vi "string2timestamp.vi"(1 "date/time string":string) -> (0 "time stamp":timestamp)   [LabVIEW 2010]
doc: "This VI convert a date/time string back to a time stamp."
uses:
  <vilib>/Utility/miscctls.llb/LVDateTimeRec.ctl
panel:
  # "This control should have data in the form:\n4/30/2004 7:48:47 PM"
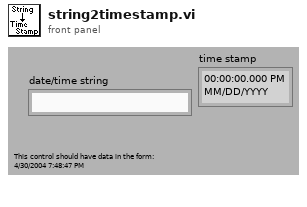
[diagram p1: front panel]
types:
  T1 = typedef "LVDateTimeRec.ctl" = cluster{"fractional second":dbl, "second":i32, "minute":i32, "hour":i32, "day of month":i32, "month":i32, "year":i32, "day of week":i32, "day of year":i32, "DST":i32}
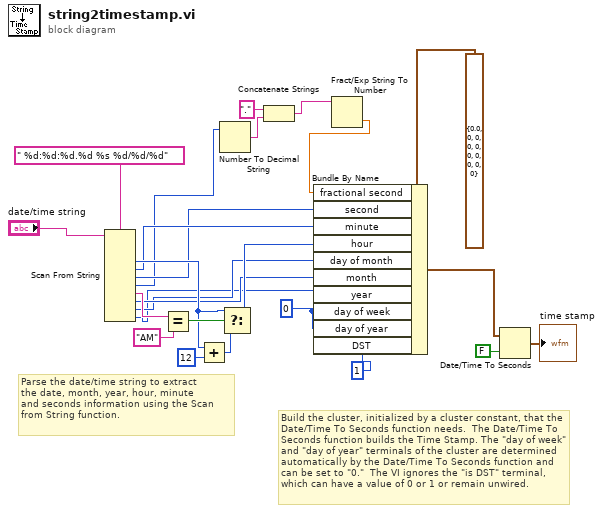
[diagram p0: block diagram]
diagram:
  w23 = 0
  # "Build the cluster, initialized by a cluster constant, that the Date/Time To Seconds function needs.  The Date/Time To Seconds function builds the Time Stamp. The \"day of week\" and \"day of year\" terminals of the cluster are determined automatically by the Date/Time To Seconds function and can be set to \"0.\"  The VI ignores the \"is DST\" terminal, which can have a value of 0 or 1 or remain unwired."
  # "Parse the date/time string to extract \nthe date, month, year, hour, minute \nand seconds information using the Scan\nfrom String function."
  n1 = Scan From String "Scan From String"(format string=" %d:%d:%d.%d %s %d/%d/%d", input string="date/time string") -> (output 1=w17:i32, output 2=w16:i32, output 3=w10:i32, output 4=w8:i32, output 5=w15:string, output 6=w14:i32, output 7=w13:i32, output 8=w12:i32)  [unwired: 10 in, 3 out]
  n2 = Equal?(x=w15, y="AM") -> (x = y?=w21:bool)
  n3 = Add(x=w17, y=12) -> (x+y=w19:i32)
  n4 = Number To Decimal String(number=w8) -> (decimal integer string=w7:string)  [unwired: 1 in]
  n5 = Select(t=w17, s=w21, f=w19) -> (s? t:f=w20:i32)
  n6 = Concatenate Strings("." ("string"), w7) -> (w5:string)
  n7 = Fract/Exp String To Number(string=w5) -> (number=w4:dbl)  [unwired: 3 in, 1 out]
  n8 = Bundle By Name(cluster=T1 {"fractional second"=0.0, "second"=0, "minute"=0, "hour"=0, "day of month"=0, "month"=0, "year"=0, "day of week"=0, "day of year"=0, "DST"=0} ("date time rec"), "fractional second"=w4, "second"=w10, "minute"=w16, "hour"=w20, "day of month"=w13, "month"=w14, "year"=w12, "day of week"=w23, "day of year"=w23, "DST"=1) -> (w9:T1)
  n9 = Date/Time To Seconds(1:FALSE ("is UTC (F)"), 2:w9) -> (0:→"time stamp":timestamp)
